vi "BCD to REG.vi"(1 "BCD Value":dbl format="%.3f") -> (0 "REG":u16[](array[numeric]))   [LabVIEW 2019, in "Userlib.lvlib"]
uses:
  Userlib.lvlib
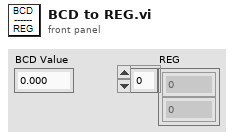
[diagram p1: front panel]
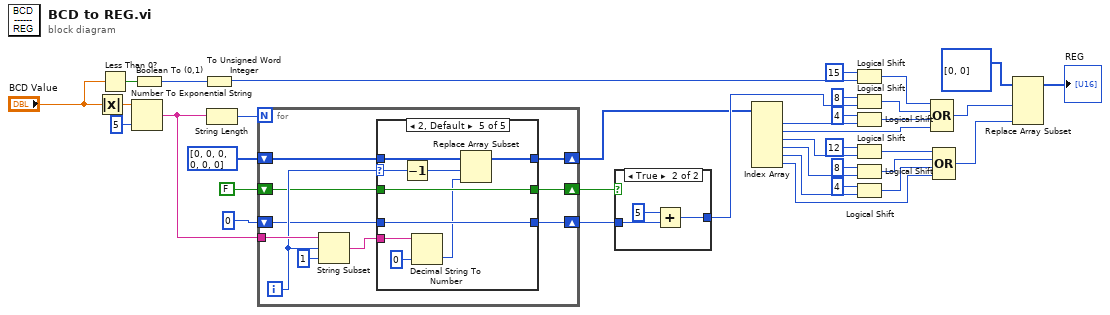
[diagram p0: block diagram]
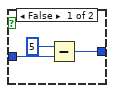
[diagram p2: hidden frame]
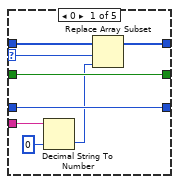
[diagram p3: hidden frame]
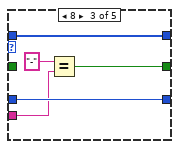
[diagram p5: hidden frame]
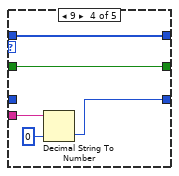
[diagram p6: hidden frame]
diagram:
  n1 = Absolute Value(x="BCD Value") -> (abs(x)=w7:dbl)
  n2 = Less Than 0?(x="BCD Value") -> (x < 0?=w5:bool)
  n3 = Number To Exponential String(number=w7, precision (6)=i16 5) -> (E-format string=w8:string)  [unwired: 2 in]
  n4 = Boolean To (0,1)(Boolean=w5) -> (0, 1=w4:i16)
  n5 = To Unsigned Word Integer(number=w4) -> (unsigned 16bit integer=w1:u16)
  n6 = String Length(string=w8) -> (length=w28:i32)
  n7 = for {
    N: w28 -> [_]
    tunnel: w8 -> [w47]
    shift-right: [w42] -> w9
    shift-left: u16[] [0, 0, 0, 0, 0, 0] ("Array") -> [w44]
    shift-right: [w39] -> w24
    shift-left: FALSE -> [w41]
    shift-right: [w38] -> w23
    shift-left: u16 0 ("offset") -> [w40]
    i -> [w45]
    n8 = String Subset(string=w47, offset (0)=w45, length (rest)=1 ("length (rest)")) -> (substring=w43:string)
    n9 = case shown="2, Default" w45 {
      selector: w45 -> [w54 _ _ _ w74]
      tunnel: w44 -> [w55 w58 w63 w68 w77]
      tunnel: w43 -> [w49 _ w61 w65 w70]
      tunnel: [w53 w58 w63 w68 w76] -> w42
      tunnel: w41 -> [w52 w57 _ w67 w73]
      tunnel: w40 -> [w51 w56 w62 _ w72]
      tunnel: [w52 w57 w59 w67 w73] -> w39
      tunnel: [w51 w56 w62 w64 w72] -> w38
      frame 0 {
        n10 = Decimal String To Number(string=w49, default (0L)=u16 0 ("offset")) -> (number=w48:u16)  [unwired: 1 in, 1 out]
        n11 = Replace Array Subset(array=w55, new element=w48, index=w54) -> (w53:u16[])
      }
      frame 1, 7 {
      }
      frame 8 {
        n12 = Equal?(x="-", y=w61) -> (x = y?=w59:bool)
      }
      frame 9 {
        n13 = Decimal String To Number(string=w65, default (0L)=u16 0 ("offset")) -> (number=w64:u16)  [unwired: 1 in, 1 out]
      }
      frame 2, Default {
        n14 = Decrement(x=w74) -> (x-1=w75:i32)
        n15 = Decimal String To Number(string=w70, default (0L)=u16 0 ("offset")) -> (number=w69:u16)  [unwired: 1 in, 1 out]
        n16 = Replace Array Subset(array=w77, new element=w69, index=w75) -> (w76:u16[])
      }
    }
  }
  n17 = case shown="True" w24 {
    tunnel: w23 -> [w79 w83]
    tunnel: [w78 w81] -> w17
    frame False {
      n18 = Subtract(x=u16 5, y=w79) -> (x-y=w78:u16)
    }
    frame True {
      n19 = Add(x=u16 5, y=w83) -> (x+y=w81:u16)
    }
  }
  n20 = Index Array(array=w9) -> (element #1=w19:u16, element #2=w18:u16, element #3=w16:u16, element #4=w15:u16, element #5=w14:u16, element #6=w13:u16)  [unwired: 6 in]
  n21 = Logical Shift(y=i16 15, x=w1) -> (x << y=w2:u16)
  n22 = Logical Shift(y=i16 8, x=w17) -> (x << y=w20:u16)
  n23 = Logical Shift(y=i16 4, x=w19) -> (x << y=w21:u16)
  n24 = Logical Shift(y=i16 12, x=w16) -> (x << y=w12:u16)
  n25 = Logical Shift(y=i16 8, x=w15) -> (x << y=w11:u16)
  n26 = Logical Shift(y=i16 4, x=w14) -> (x << y=w10:u16)
  n27 = Compound Arithmetic op=OR(w2, w20, w21, w18) -> (w31:u16)
  n28 = Compound Arithmetic op=OR(w12, w11, w10, w13) -> (w32:u16)
  n29 = Replace Array Subset(array=u16[] [0, 0] ("appended array"), new element #1=w31, new element #2=w32) -> (→"REG":u16[])  [unwired: 2 in]
